vi "test_Create MetaData Channel_array enumerated list.vi"(8 "error in (no error)":errorcluster, 11 "TestCase in":refnum<class "Instrument Addon Scripting API Channels Unit Tests.lvclass">) -> (0 "error out":errorcluster, 3 "TestCase out":refnum<class "Instrument Addon Scripting API Channels Unit Tests.lvclass">)   [LabVIEW 2018, in "Instrument Addon Scripting API Channels Unit Tests.lvclass"]
uses:
  Instrument Addon Scripting API Channels Unit Tests.lvclass
  Addon/Addon Shared/Types/FG Control.ctl
  APIs/Scripting API/TypeDefs/Array Enumerated List Settings.ctl
  APIs/Scripting API/TypeDefs/Array Element.ctl
  Instrument Addon Scripting API Channels Unit Tests.lvclass/Instrument Addon Scripting API Channels Unit Tests.ctl
  Addon/Addon Shared/SubVIs/Constants.vi
  <vilib>/NI Veristand/Custom Device Tools/Custom Device Utility Library/NI VeriStand - Search for Item by Name.vi
  APIs/Scripting API/Channels/Create MetaData Channel - Array - Enumerated List.vi
  <vilib>/NI Veristand/Custom Device Tools/Custom Device Utility Library/NI VeriStand - Search for Item by GUID.vi
  <vilib>/NI Veristand/Custom Device API/NI VeriStand - Get Item Property.vi
  <vilib>/NI Veristand/Custom Device API/Get Item Property (U32).vi
  <vilib>/NI Veristand/Custom Device API/Get Item Property (String Array).vi
  <vilib>/NI Veristand/Custom Device API/Get Item Property (String).vi
  <vilib>/NI Veristand/Custom Device API/NI VeriStand - Set Item Property.vi
  <vilib>/NI Veristand/Custom Device API/Set Item Property (U32).vi
  <vilib>/NI Veristand/Custom Device API/Set Item Property (String Array).vi
  <vilib>/NI Veristand/Custom Device API/NI VeriStand - Get Item Children.vi
  Addon/Addon Shared/SubVIs/Set Channel Value Table.vi
  <vilib>/NI Veristand/Custom Device API/Set Item Property (String).vi
  <vilib>/addons/_JKI Toolkits/VI Tester/TestCase.llb/TestCase.lvclass
  Instrument Addon Scripting API Test Assets/Instrument Addon Scripting API Test Assets.lvclass
  <vilib>/NI Veristand/Custom Device Tools/Custom Device Utility Library/Custom Device Utility Library.lvlib
  Addon/Addon Shared/Instrument Addon Shared.lvlib
  APIs/Scripting API/Instrument Addon Scripting API.lvlib
  C:/Program Files (x86)/National Instruments/LabVIEW 2018/vi.lib/addons/_JKI Toolkits/VI Tester/TestCase.llb/TestCase.lvclass
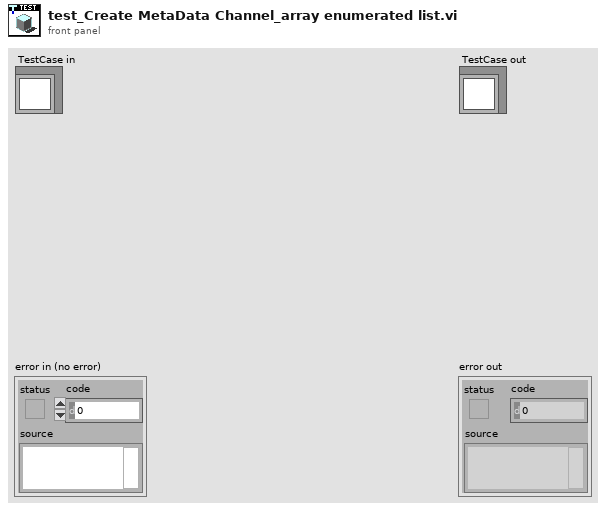
[diagram p1: front panel]
types:
  T1 = typedef "Instrument Addon Shared.lvlib/FG Control.ctl" = enum16{"Get", "Set"}
  T2 = typedef "Instrument Addon Scripting API.lvlib/Array Enumerated List Settings.ctl" = cluster{"Elements":T3[], "Enumerated List":string[], "Delimiter":string}
  T3 = typedef "Instrument Addon Scripting API.lvlib/Array Element.ctl" = cluster{"Name":string, "Default Value":dbl, "Units":string}
  T4 = typedef "Custom Device API.lvlib/Custom Device Item Ref.ctl" = u64
  T5 = typedef "Instrument Addon Shared.lvlib/MetaData Parameters.ctl" = cluster{"Data Type":T6, "Channel Type":T7, "List":string[], "Format String":string, "Type":T8, "Delimiter":string, "Endian":T9}
  T6 = typedef "Instrument Addon Shared.lvlib/Protocol Data Type.ctl" = enum16{"Single Channel", "Array"}
  T7 = typedef "Instrument Addon Shared.lvlib/Metadata Channel Type.ctl" = enum16{"Enumerated List", "Format", "Type Cast"}
  T8 = typedef "Instrument Addon Shared.lvlib/Type Cast Type.ctl" = enum16{"DBL", "SGL", "U64", "U32", "U16", "U8", "I64", "I32", "I16", "I8"}
  T9 = typedef "Instrument Addon Shared.lvlib/Endian.ctl" = enum16{"Native", "Little", "Big"}
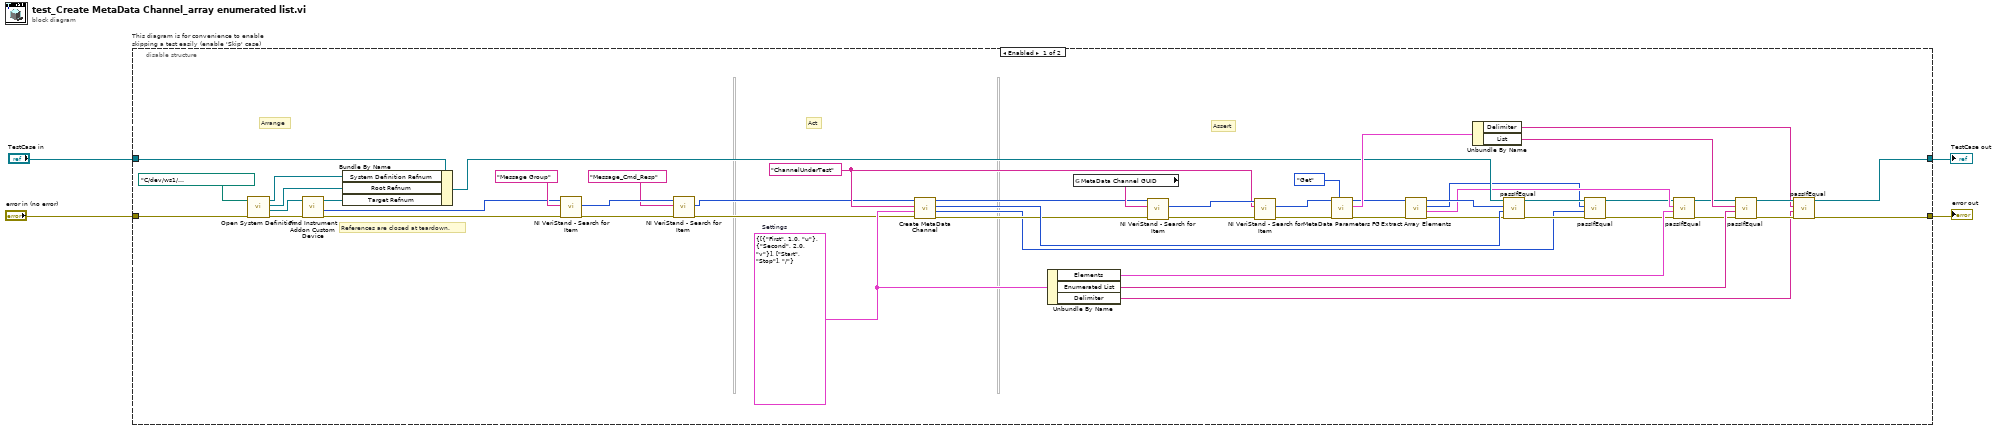
[diagram p0: block diagram]
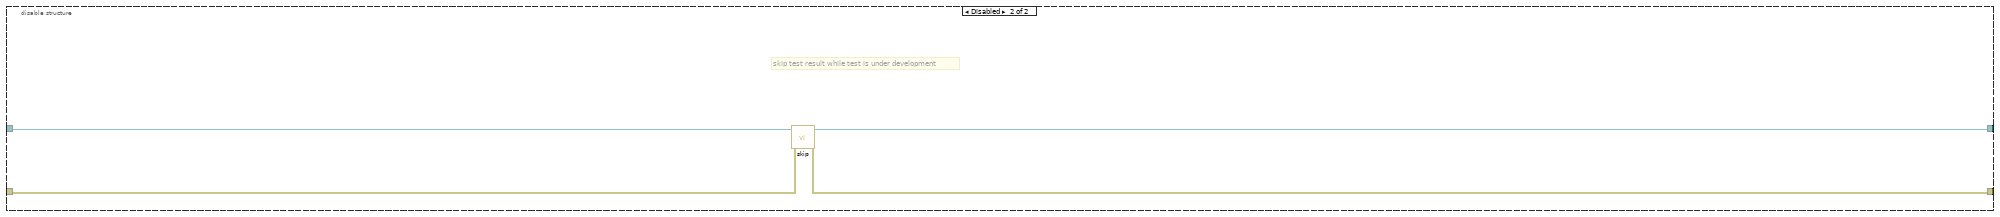
[diagram p2: hidden frame]
diagram:
  n1 = disable-structure "This diagram is for convenience to enable skipping a test easily (enable 'Skip' case)" shown="Enabled" {
    disable-tunnel: "TestCase in" -> [w36 w59]
    disable-tunnel: [w28 w57] -> w1
    disable-tunnel: [w27 w58] -> w3
    disable-tunnel: "error in (no error)" -> [w55 w56]
    frame Enabled {
      w31 = T2 {"Elements"=[{"Name"="First", "Default Value"=1.0, "Units"="u"}, {"Name"="Second", "Default Value"=2.0, "Units"="v"}], "Enumerated List"=["Start", "Stop"], "Delimiter"="/"}  # Settings
      w35 = "ChannelUnderTest" ("Name")
      # "References are closed at teardown."
      # "Assert"
      # "Act"
      # "Arrange"
      n2 = call "Open System Definition.vi"("error in (no error)"=w55, "System Definition File"=path "C:/dev/ws1/niveristand-instrument-addon-custom-device/Source/Tests/Unit Tests/Scripting API/Instrument Addon Scripting API Channels Unit Tests/Assets/MetaData Channels/IACD_channels.nivssdf") -> ("error out"=w53:errorcluster, "Target Refnum"=w54:refnum<k24>, "Root Refnum"=w39:refnum<k24>, "System Definition Refnum"=w38:refnum<k24>)  [unwired: 6 in]
      n3 = call "Find Instrument Addon Custom Device.vi"("error in"=w53, "target in"=w54) -> ("error out"=w13:errorcluster, "NodeID"=w15:u64, "target out"=w40:refnum<k24>)  [unwired: 7 in]
      n4 = Bundle By Name(cluster=w36, "System Definition Refnum"=w38, "Root Refnum"=w39, "Target Refnum"=w40) -> (w37:refnum<class "Instrument Addon Scripting API Channels Unit Tests.lvclass">)
      n5 = call-poly <vilib>:"NI VeriStand - Search for Item.vi"("error in"=w13, "Item Name"="Message Group", "Section Ref in"=w15) -> ("error out"=w16:errorcluster, "Item Ref"=w18:T4)  [unwired: 5 in, 2 out]
      n6 = call-poly <vilib>:"NI VeriStand - Search for Item.vi"("error in"=w16, "Item Name"="Message_Cmd_Resp", "Section Ref in"=w18) -> ("error out"=w12:errorcluster, "Item Ref"=w14:T4)  [unwired: 5 in, 2 out]
      n7 = call-poly "Create MetaData Channel.vi"("Error In"=w12, "Settings"=w31, "Name"=w35, "Message Refnum In"=w14) -> ("Error Out"=w32:errorcluster, "Channel Refnums"=w5:T4[], "Array Refnum"=w33:T4, "Message Refnum Out"=w34:T4)  [unwired: 4 in]
      n8 = Unbundle By Name(w31) -> ("Elements"=w24:T3[], "Enumerated List"=w41:string[], "Delimiter"=w30:string)
      n9 = global read "Constants.vi" "MetaData Channel GUID"() -> (w51:string)
      n10 = call-poly <vilib>:"NI VeriStand - Search for Item.vi"("error in"=w32, "Item GUID"=w51, "Section Ref in"=w34) -> ("error out"=w49:errorcluster, "Item Ref"=w50:T4)  [unwired: 5 in, 2 out]
      n11 = call-poly <vilib>:"NI VeriStand - Search for Item.vi"("error in"=w49, "Item Name"=w35, "Section Ref in"=w50) -> ("error out"=w48:errorcluster, "Item Ref"=w47:T4)  [unwired: 5 in, 2 out]
      n12 = call "MetaData Parameters FG.vi"("Action"=FG_Control."Get", "error in (no error)"=w48, "Item Ref in"=w47) -> ("error out"=w23:errorcluster, "MetaData Parameters"=w45:T5, "Item Ref out"=w22:T4)  [unwired: 6 in]
      n13 = call "Extract Array Elements.vi"("error in (no error)"=w23, "array reference in"=w22) -> ("error out"=w21:errorcluster, "elements"=w11:T3[], "channel refnums"=w6:T4[], "array reference out"=w20:T4)  [unwired: 6 in]
      n14 = Unbundle By Name(w45) -> ("Delimiter"=w29:string, "List"=w42:string[])
      n15 = call-dynamic "passIfEqual.vi"("error in (no error)"=w21, "y"=w33, "x"=w20, "TestCase in"=w37) -> ("error out"=w9:errorcluster, "TestCase out"=w10:refnum<class "Instrument Addon Scripting API Channels Unit Tests.lvclass">)  [unwired: 6 in]
      n16 = call-dynamic "passIfEqual.vi"("error in (no error)"=w9, "y"=w5, "x"=w6, "TestCase in"=w10) -> ("error out"=w8:errorcluster, "TestCase out"=w7:refnum<class "Instrument Addon Scripting API Channels Unit Tests.lvclass">)  [unwired: 6 in]
      n17 = call-dynamic "passIfEqual.vi"("error in (no error)"=w8, "y"=w24, "x"=w11, "TestCase in"=w7) -> ("error out"=w25:errorcluster, "TestCase out"=w26:refnum<class "Instrument Addon Scripting API Channels Unit Tests.lvclass">)  [unwired: 6 in]
      n18 = call-dynamic "passIfEqual.vi"("error in (no error)"=w25, "y"=w41, "x"=w42, "TestCase in"=w26) -> ("error out"=w44:errorcluster, "TestCase out"=w43:refnum<class "Instrument Addon Scripting API Channels Unit Tests.lvclass">)  [unwired: 6 in]
      n19 = call-dynamic "passIfEqual.vi"("error in (no error)"=w44, "y"=w30, "x"=w29, "TestCase in"=w43) -> ("error out"=w27:errorcluster, "TestCase out"=w28:refnum<class "Instrument Addon Scripting API Channels Unit Tests.lvclass">)  [unwired: 6 in]
    }
    frame Disabled {
      # "skip test result while test is under development"
      n20 = call <vilib>:"skip.vi"("error in (no error)"=w56, "TestCase in"=w59) -> ("error out"=w58:errorcluster, "TestCase out"=w57:refnum<class "Instrument Addon Scripting API Channels Unit Tests.lvclass">)  [unwired: 8 in]
    }
  }
  "error out" <- w3
  "TestCase out" <- w1
